vi "Prog7.vi"() -> ()   [LabVIEW 2021]
panel:
  out "x = y? 3":bool[](array[boolean])
  out "x > y?":bool
  out "x = y? 2":bool
  out "x = y?":bool
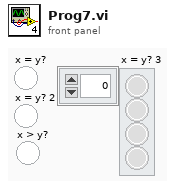
[diagram p1: front panel]
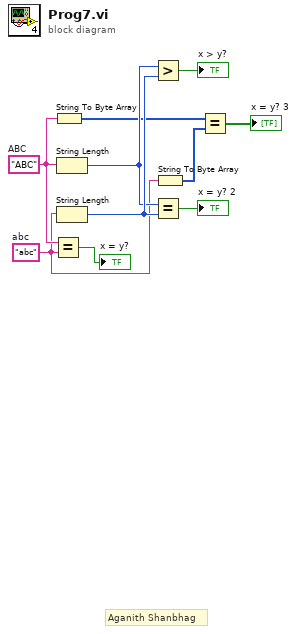
[diagram p0: block diagram]
diagram:
  w3 = "abc"  # abc
  w5 = "ABC"  # ABC
  # "Aganith Shanbhag"
  n1 = Equal?(x=w5, y=w3) -> (x = y?=→"x = y?":bool)
  n2 = String To Byte Array(string=w5) -> (unsigned byte array=w4:u8[])
  n3 = String Length(string=w5) -> (length=w8:i32)
  n4 = String Length(string=w3) -> (length=w9:i32)
  n5 = Greater?(x=w8, y=w9) -> (0:→"x > y?":bool)
  n6 = Equal?(x=w8, y=w9) -> (x = y?=→"x = y? 2":bool)
  n7 = String To Byte Array(string=w3) -> (unsigned byte array=w2:u8[])
  n8 = Equal?(x=w4, y=w2) -> (x = y?=→"x = y? 3":bool[])
